vi "dfd_Lattice AR Normalization (Norm).vi"(7 "scale type":T1, 10 "coefficients k":dbl[](array[numeric]) format="%.2f", 11 "x":dbl[](array[numeric])) -> (2 "norm":dbl[](array[numeric]) format="%.2f", 3 "y":dbl[](array[numeric]))   [LabVIEW 2017, in "NI_DigFilter_FXP.lvlib"]
uses:
  <vilib>/addons/Digital Filter Design/NI_DigFilter_FXP.lvlib
  <vilib>/addons/Digital Filter Design/_Objects.llb/DFD Coef Norm Type.ctl
  <vilib>/addons/Digital Filter Design/NI_DigFilterLicensed.lvlib
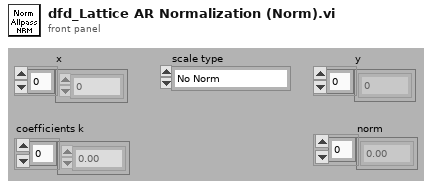
[diagram p1: front panel]
types:
  T1 = typedef "NI_DigFilterLicensed.lvlib/DFD Coef Norm Type.ctl" = enum16{"No Norm", "Time Domain 1-Norm", "Time Domain 2-Norm", "Time Domain Inf-Norm"}
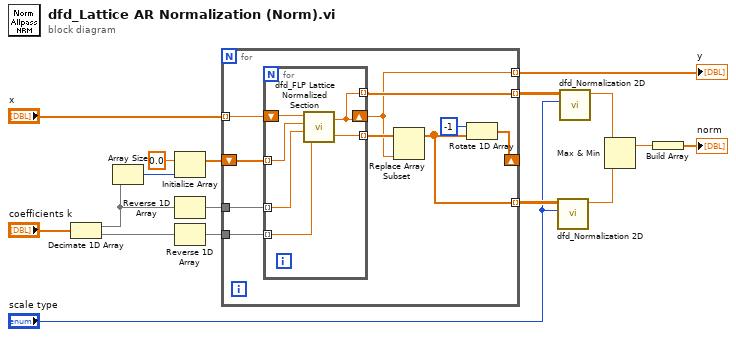
[diagram p0: block diagram]
diagram:
  n1 = Decimate 1D Array("coefficients k") -> (w3:dbl[], w2:dbl[])
  n2 = Array Size(array=w3) -> (size(s)=w16:i32)
  n3 = Initialize Array(0.0 ("element"), w16) -> (w17:dbl[])
  n4 = Reverse 1D Array(array=w3) -> (reversed array=w15:dbl[])
  n5 = Reverse 1D Array(array=w2) -> (reversed array=w1:dbl[])
  n6 = for {
    tunnel: w15 -> [w27]
    shift-right: [w26] -> _
    shift-left: w17 -> [w25]
    tunnel: [w19] -> w10 mode=indexing
    tunnel: [w24] -> w11 mode=indexing
    tunnel: "x" -> [w22] mode=indexing
    tunnel: [w20] -> w5 mode=indexing
    tunnel: w1 -> [w21]
    n7 = for {
      shift-right: [w30] -> w20
      shift-left: w22 -> [w29]
      tunnel: w25 -> [w33] mode=indexing
      tunnel: w27 -> [w32] mode=indexing
      tunnel: [w31] -> w23 mode=indexing
      tunnel: [w30] -> w24 mode=indexing
      tunnel: w21 -> [w28] mode=indexing
      n8 = call <vilib>:"dfd_FLP Lattice Normalized Section.vi"("^k(m)"=w28, "k(m)"=w32, "w(m-1)"=w33, "x(m)"=w29) -> ("w(m)"=w31:dbl, "x(m-1)"=w30:dbl)
    }
    n9 = Replace Array Subset(array=w23, new element=w20) -> (w19:dbl[])  [unwired: 1 in]
    n10 = Rotate 1D Array(1:w19, 2:-1 ("n")) -> (0:w26:dbl[])
  }
  "y" <- w5
  n11 = call <vilib>:"dfd_Normalization 2D.vi"("scale type"="scale type", "2D Array (col-major)"=w10) -> ("max norm"=w8:dbl)  [unwired: 9 out]
  n12 = call <vilib>:"dfd_Normalization 2D.vi"("scale type"="scale type", "2D Array (col-major)"=w11) -> ("max norm"=w7:dbl)  [unwired: 9 out]
  n13 = Max & Min(x=w7, y=w8) -> (max(x,y)=w6:dbl)  [unwired: 1 out]
  n14 = Build Array(w6) -> (→"norm":dbl[])
